vi "Verify Hardware Custom Devices Exist.vi"(8 "error in (no error)":errorcluster, 11 "Routing and Faulting Custom Device Ref in":T1 format="%.0x") -> (0 "error out":errorcluster, 3 "Routing and Faulting Custom Device Ref out":T1 format="%.0x")   [LabVIEW 2017]
uses:
  <vilib>/NI Veristand/Custom Device API/Custom Device Item Ref.ctl
  Routing and Faulting Scripting.lvlib
  <vilib>/NI Veristand/Custom Device API/Custom Device API.lvlib
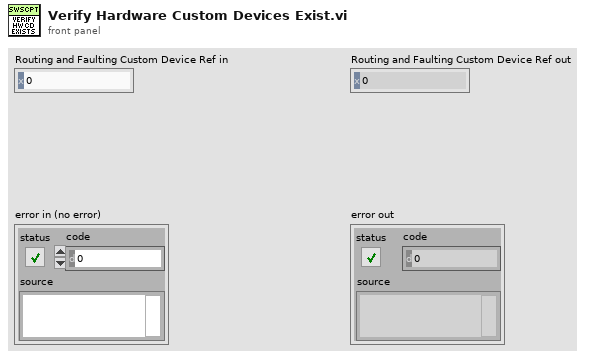
[diagram p1: front panel]
types:
  T1 = typedef "Custom Device API.lvlib/Custom Device Item Ref.ctl" = u64
  T2 = typedef "Routing and Faulting Scripting.lvlib/Module Connection Information.ctl" = cluster{"Module Path":string, "Model":string, "Possible Connections":T3[]}
  T3 = typedef "Routing and Faulting Hardware API.lvlib/Possible Connections for Endpoint.ctl" = cluster{"Source":string, "Destinations":string[]}
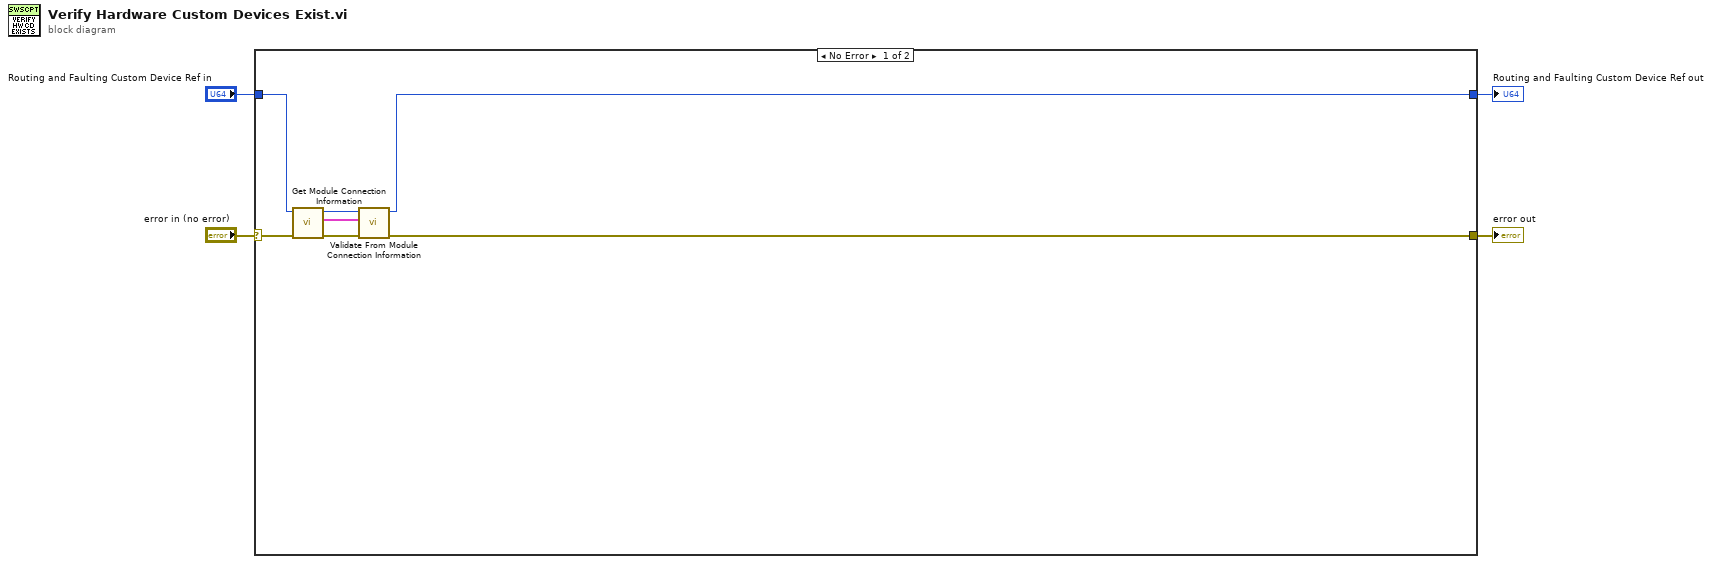
[diagram p0: block diagram]
diagram:
  n1 = case shown="No Error" "error in (no error)" {
    selector: "error in (no error)" -> [w11 w13]
    tunnel: "Routing and Faulting Custom Device Ref in" -> [w10 w12]
    tunnel: [w7 w13] -> w3
    tunnel: [w5 w12] -> w1
    frame No Error {
      n2 = call "Get Module Connection Information.vi"("error in (no error)"=w11, "Routing and Faulting Custom Device Ref in"=w10) -> ("error out"=w9:errorcluster, "Module Connection Information"=w8:T2[], "Routing and Faulting Custom Device Ref out"=w6:T1)  [unwired: 7 in]
      n3 = call "Validate From Module Connection Information.vi"("error in (no error)"=w9, "Module Connection Information"=w8, "Routing and Faulting Custom Device Ref in"=w6) -> ("error out"=w7:errorcluster, "Routing and Faulting Custom Device Ref out"=w5:T1)  [unwired: 7 in]
    }
    frame Error {
    }
  }
  "Routing and Faulting Custom Device Ref out" <- w1
  "error out" <- w3
